vi "Prepare.vi"(8 "error in":errorcluster, 10 "Iterator Settings":T1={"Prepare timeout (ms)"=200, "Iterate timeout (ms)"=50, "Conclude timeout (ms)"=200, "Iterate period (ms)"=200, "Number of iterations"=5, "Time before stop (ms)"=5, "Active Stop Conditions"={"Number of Iterations"=FALSE, "Time Elapsed"=FALSE, "Iteration Result"=FALSE}, "Prepare Msg"=refnum, "Iterate Msg"=refnum, "Conclude Msg"=refnum, "Iterations End Report"=refnum, "Message Priority (Normal)"=enum."Normal"}, 11 "Iterator Actor in":refnum<class "Iterator Actor.lvclass">) -> (0 "error out":errorcluster, 2 "Reply":bool, 3 "Iterator Actor out":refnum<class "Iterator Actor.lvclass">)   [LabVIEW 2023, in "Iterator Actor.lvlib" / "Iterator Actor.lvclass"]
doc: "Calls the Prepare method of the Client and receives its responce."
uses:
  Iterator Actor.lvclass
  Abstract Iterator Actor/Iterator Settings.ctl
  Abstract Iterator Actor Messages/Iterator Report Iterations End Msg/Iterator Report Iterations End Msg.lvclass
  <vilib>/ActorFramework/Message/Message.lvclass
  Abstract Iterator Actor/Active Stop Conditions.ctl
  <vilib>/ActorFramework/Message Enqueuer/Message Priority.ctl
  C:/Projects/Iterator Actor/Abstract Iterator Actor/Abstract Iterator Actor.lvclass
  C:/Program Files/National Instruments/LabVIEW 2023/vi.lib/ActorFramework/Actor/Actor.lvclass
  Abstract Iterator Actor/Abstract Iterator Actor.lvclass/Abstract Iterator Actor.ctl
  <vilib>/ActorFramework/Actor/Actor.lvclass/Actor.ctl
  Iterator Actor Messages/Iterator Reply Msg/Iterator Reply Msg.lvclass
  Abstract Iterator Actor/Read Stop Iterate Notifier.vi
  <vilib>/Utility/error.llb/Error Cluster From Error Code.vi
  <vilib>/ErrorRing/Error Ring.xnode
  Iterator Actor.lvclass/Iterator Actor.ctl
  <vilib>/ActorFramework/Actor/Actor.lvclass
  Abstract Iterator Actor/Abstract Iterator Actor.lvclass
  <vilib>/ActorFramework/Message Enqueuer/Message Enqueuer.lvclass
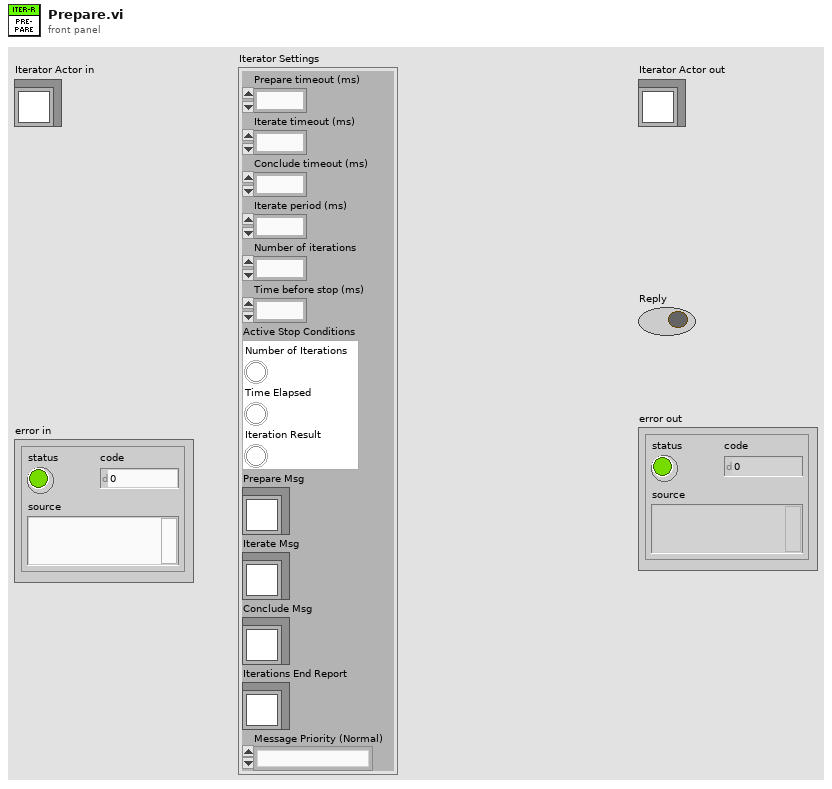
[diagram p1: front panel]
types:
  T1 = typedef "Iterator Actor.lvlib/Abstract Iterator Actor.lvclass/Iterator Settings.ctl" = cluster{"Prepare timeout (ms)":i32, "Iterate timeout (ms)":i32, "Conclude timeout (ms)":i32, "Iterate period (ms)":i32, "Number of iterations":i32, "Time before stop (ms)":i32, "Active Stop Conditions":T2, "Prepare Msg":refnum<class "Message.lvclass">, "Iterate Msg":refnum<class "Message.lvclass">, "Conclude Msg":refnum<class "Message.lvclass">, "Iterations End Report":refnum<class "Iterator Report Iterations End Msg.lvclass">, "Message Priority (Normal)":T3}
  T2 = typedef "Iterator Actor.lvlib/Abstract Iterator Actor.lvclass/Active Stop Conditions.ctl" = cluster{"Number of Iterations":bool, "Time Elapsed":bool, "Iteration Result":bool}
  T3 = typedef "Actor Framework.lvlib/Message Enqueuer.lvclass/Message Priority.ctl" = enum16{"Low", "Normal", "High"}
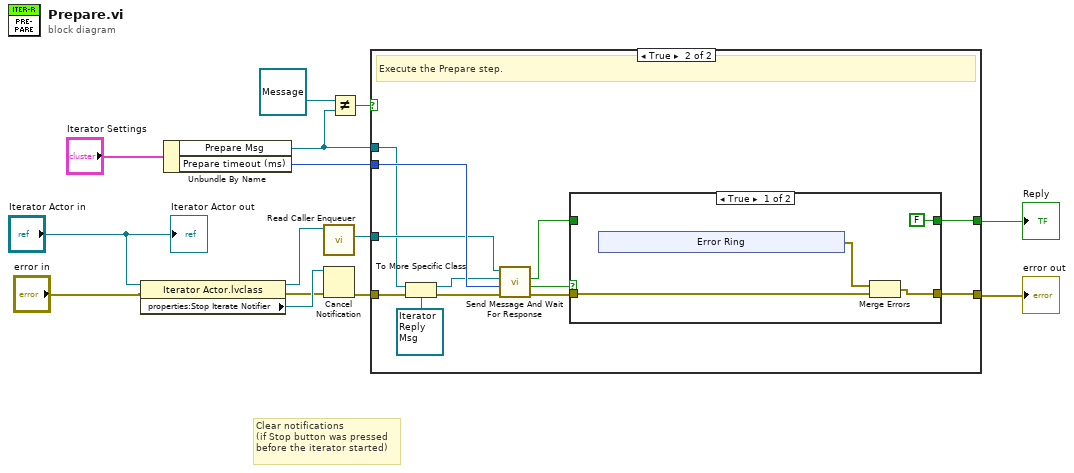
[diagram p0: block diagram]
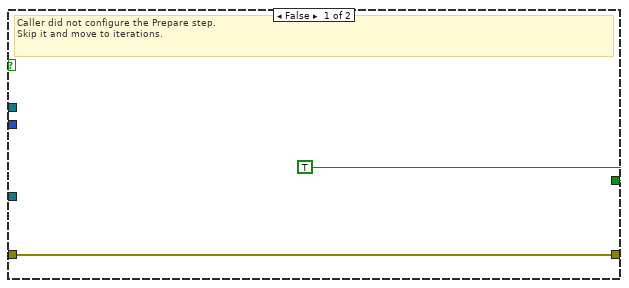
[diagram p2: hidden frame]
diagram:
  # "Clear notifications\n(if Stop button was pressed\nbefore the iterator started)"
  n1 = property class="Iterator Actor.lvclass"(reference="Iterator Actor in", error in="error in") -> (reference out=w1:refnum<class "Iterator Actor.lvclass">, error out=w4:errorcluster, "properties:Stop Iterate Notifier"=w6:refnum<notifier>)
  n2 = Unbundle By Name("Iterator Settings") -> ("Prepare Msg"=w2:refnum<class "Message.lvclass">, "Prepare timeout (ms)"=w14:i32)
  n3 = call <vilib>:"Read Caller Enqueuer.vi"("Actor"=w1) -> ("Caller Enqueuer"=w8:refnum<class "Message Enqueuer.lvclass">)  [unwired: 10 in]
  n4 = Cancel Notification(0:w6, 3:w4) -> (11:w10:errorcluster)  [unwired: 2 out]
  n5 = Not Equal?(x=refnum<class "Message.lvclass"> refnum ("Prepare Msg"), y=w2) -> (x != y?=w9:bool)
  n6 = case shown="True" w9 {
    tunnel: w14 -> [_ w28]
    tunnel: w2 -> [_ w23]
    tunnel: [TRUE w18] -> w12
    tunnel: [w15 w17] -> w11
    tunnel: w8 -> [_ w27]
    tunnel: w10 -> [w15 w26]
    frame False {
      # "Caller did not configure the Prepare step.\nSkip it and move to iterations."
    }
    frame True {
      # "Execute the Prepare step."
      n7 = To More Specific Class(target class=refnum<class "Iterator Reply Msg.lvclass"> refnum ("Prepare Msg"), reference=w23, error in=w26) -> (specific class reference=w22:refnum<class "Iterator Reply Msg.lvclass">, error out=w25:errorcluster)
      n8 = call "Send Message And Wait For Response.vi"("error in (no error)"=w25, "timeout in ms (-1)"=w28, "Original Message"=w22, "Message Enqueuer in"=w27) -> ("error out"=w21:errorcluster, "timed out?"=w20:bool, "Reply"=w19:bool)  [unwired: 4 in, 1 out]
      n9 = case shown="True" w20 {
        tunnel: w21 -> [w32 w38]
        tunnel: [w31 w38] -> w17
        tunnel: w19 -> [_ w37]
        tunnel: [FALSE ("Reply") w37] -> w18
        frame True {
          n10 = xnode "Error Ring"() -> ("error out"=w30:errorcluster)
          n11 = Merge Errors(w30, w32) -> (w31:errorcluster)
        }
        frame False {
        }
      }
    }
  }
  "Reply" <- w12
  "error out" <- w11
  "Iterator Actor out" <- "Iterator Actor in"
